vi "TW Update Library Name.vi"(6 "Update Folder Name":bool, 8 "error in (no error)":errorcluster, 9 "Replace Subname":string="Template", 10 "New Subname":string, 11 "Library in":refnum<vi>) -> (0 "error out":errorcluster)   [LabVIEW 2021, in "Plugin Generator.lvlib"]
uses:
  Plugin Generator.lvlib
  <vilib>/Utility/EditLVLibs/Edit LVLibs.lvlib
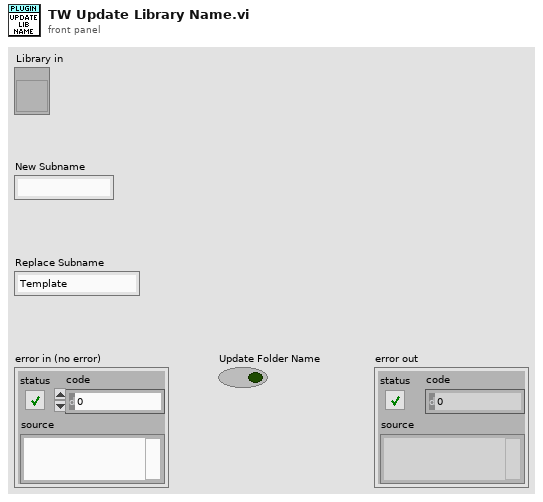
[diagram p1: front panel]
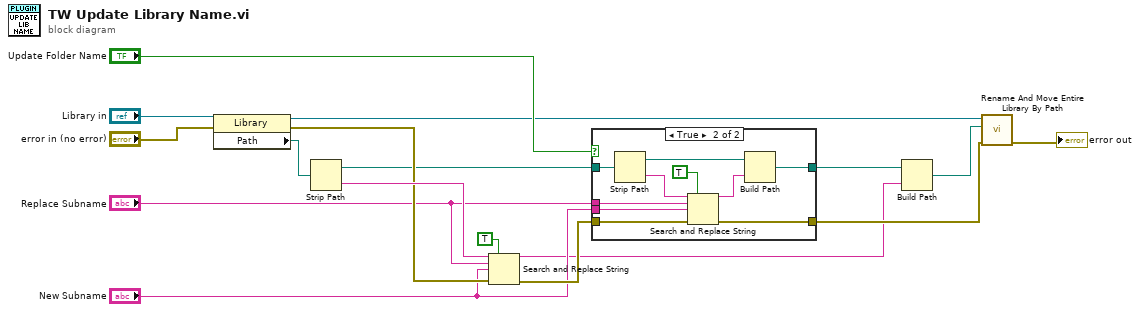
[diagram p0: block diagram]
diagram:
  n1 = property class="Library"(reference="Library in", error in="error in (no error)") -> (reference out=w3:refnum<vi>, error out=w13:errorcluster, "Path"=w2:path)
  n2 = Strip Path(path=w2) -> (stripped path=w10:path, name=w17:string)
  n3 = Search and Replace String(replace all?=TRUE ("replace all? (F)"), input string=w17, search string="Replace Subname", replace string="New Subname", error in=w13) -> (result string=w8:string, error out=w14:errorcluster)  [unwired: 3 in, 2 out]
  n4 = case shown="True" "Update Folder Name" {
    tunnel: [w19 w29] -> w7
    tunnel: w10 -> [w19 w28]
    tunnel: "Replace Subname" -> [_ w23]
    tunnel: "New Subname" -> [_ w22]
    tunnel: w14 -> [w18 w21]
    tunnel: [w18 w20] -> w15
    frame False {
    }
    frame True {
      n5 = Strip Path(path=w28) -> (stripped path=w27:path, name=w25:string)
      n6 = Search and Replace String(replace all?=TRUE ("replace all? (F)"), input string=w25, search string=w23, replace string=w22, error in=w21) -> (result string=w24:string, error out=w20:errorcluster)  [unwired: 3 in, 2 out]
      n7 = Build Path(base path=w27, name or relative path=w24) -> (appended path=w29:path)
    }
  }
  n8 = Build Path(base path=w7, name or relative path=w8) -> (appended path=w4:path)
  n9 = call <vilib>:"Rename And Move Entire Library By Path.vi"("error in (no error)"=w15, "New library path"=w4, "Library ref in"=w3) -> ("error out"=→"error out":errorcluster)  [unwired: 7 in, 1 out]
